vi "enableServoDefaultPosition.vi"(1 "enable bit":u8=1 max=15 step=1) -> ()   [LabVIEW 2012]
uses:
  GlobalSerial.vi
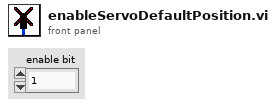
[diagram p1: front panel]
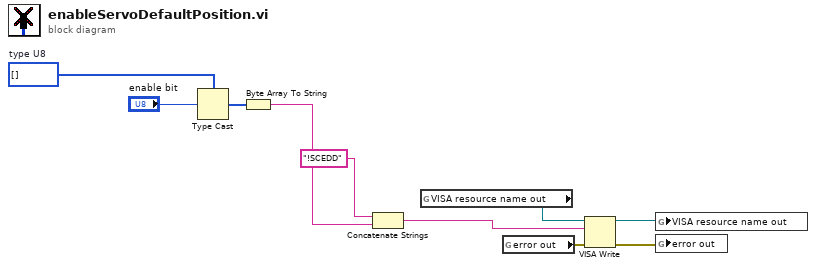
[diagram p0: block diagram]
diagram:
  w6 = u8[] []  # type U8
  n1 = Type Cast(type=w6, x="enable bit") -> (*(type *) &x=w8:u8[])
  n2 = Byte Array To String(unsigned byte array=w8) -> (string=w9:string)
  n3 = Concatenate Strings("!SCEDD" ("string"), w9) -> (w5:string)
  n4 = global read "GlobalSerial.vi" "VISA resource name out"() -> (w2:refnum<visa-resource-name>)
  n5 = global read "GlobalSerial.vi" "error out"() -> (w4:errorcluster)
  n6 = VISA Write(VISA resource name=w2, write buffer=w5, error in (no error)=w4) -> (VISA resource name out=w1:refnum<visa-resource-name>, error out=w3:errorcluster)  [unwired: 1 out]
  n7 = global write "GlobalSerial.vi" "VISA resource name out"(w1) -> ()
  n8 = global write "GlobalSerial.vi" "error out"(w3) -> ()
